vi "Select STD.vi"(8 "에러 입력(에러 없음)":errorcluster, 11 "ItemNames":string[][](array[string])) -> (0 "에러 출력":errorcluster)   [LabVIEW 2020]
uses:
  Controls/Cmd_Select Setting.ctl
  Controls/Cmd_Read Query.ctl
  Controls/Clst_Query Info.ctl
  Variables/Global_Cal STD.vi
  <vilib>/addons/database/NI_Database_API.lvlib
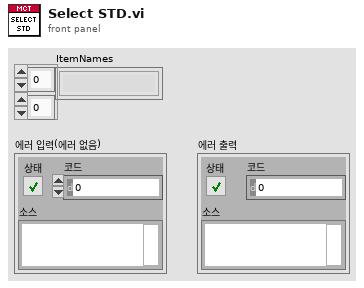
[diagram p1: front panel]
types:
  T1 = typedef "Cmd_Select Setting.ctl" = enum16{"STD Setting"}
  T2 = typedef "NI_Database_API.lvlib/Conn ObjectReference.ctl" = refnum<k1>
  T3 = typedef "Clst_Query Info.ctl" = cluster{"사번":string, "등록번호":string, "업체명":string, "세부분류코드":string, "형식":string, "기기번호":string, "FUNC":string, "FUNC_EXT":string, "옵션":string, "추가문자열":string, "일자":string, "배열 1":string[], "배열 2":string[], "항목명":string, "문자열":string, "이름":string}
  T4 = typedef "Cmd_Read Query.ctl" = enum16{"교정자 이름 얻기", "인증교정자 얻기", "기술책임자 얻기", "기책부책 얻기", "등록번호 얻기", "등록정보 얻기", "업체정보 얻기", "교정일자(CAMAS) 얻기", "교정일자(CALSTD) 얻기", "교정환경 얻기", "교정절차서 목록 얻기", "교정절차서명 얻기", "교정절차 목록얻기", "교정절차 얻기", "PROC 교정절차 얻기", "PROC SPEC 얻기", "교정절차(Func별) 얻기", "교정절차(Func_ext별) 얻기", "기관코드 얻기", "교정기능(세부분류) 얻기", "교정기능(모델) 얻기", "교정기능 목록 얻기", "교정기능 명칭 얻기", "교정기능 항목명칭 얻기", "DB (사용기준기) 얻기", "DB (기준기이름) 얻기", "DB (기준기이름목록) 얻기", "DB (기준기목록) 얻기", "DB (기준기값) 얻기", "DB (CMC) 얻기", "DB (FUNC) 얻기", "DB (CALNAME) 얻기", "DB (STDNAME) 얻기", "DB (SPEC) 얻기", "모델(항목전체) 얻기", "모델(최대범위) 얻기", "모델(최소범위) 얻기", "모델(최대최소) 얻기", "모델(범위조건) 얻기", "모델(등록요청) 얻기", "모델(형식별) 얻기", "모델(조건별) 얻기", "모델(모델검색) 얻기", "세부분류 목록 얻기", "기준기등록리스트 얻기", "STD Cal Date Check", "DB등록일자 얻기", "적용항목 얻기", "기타정보 얻기", "기준기요청 얻기", "서버버전 얻기"}
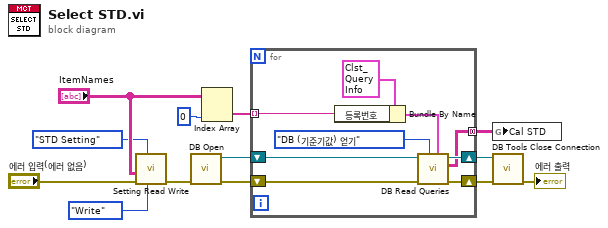
[diagram p0: block diagram]
diagram:
  n1 = call "Setting Read Write.vi"("Read/Write"=enum16{"Read", "Write"}."Write", "Select"=Cmd_Select_Setting."STD Setting", "error in (no error)"="에러 입력(에러 없음)", "Data in"="ItemNames") -> ("error out"=w10:errorcluster)  [unwired: 6 in, 1 out]
  n2 = call "DB Open.vi"("에러 입력"=w10) -> ("에러 출력"=w3:errorcluster, "참조 번호 출력"=w4:T2)  [unwired: 9 in]
  n3 = Index Array(array="ItemNames", index (col)=0 ("비활성화된 인덱스 (열)")) -> (element=w2:string[])  [unwired: 1 in]
  n4 = for {
    tunnel: w2 -> [w16] mode=indexing
    shift-right: [w20] -> w6
    shift-left: w3 -> [w22]
    shift-right: [w15] -> w5
    shift-left: w4 -> [w21]
    tunnel: [w14] -> w8 mode=concatenating
    n5 = Bundle By Name(cluster=T3 {"사번"="", "등록번호"="", "업체명"="", "세부분류코드"="", "형식"="", "기기번호"="", "FUNC"="", "FUNC_EXT"="", "옵션"="", "추가문자열"="", "일자"="", "배열 1"=[], "배열 2"=[], "항목명"="", "문자열"="", "이름"=""} ("Query info"), "등록번호"=w16) -> (w18:T3)
    n6 = call "DB Read Queries.vi"("Query info"=w18, "Query Command"=Cmd_Read_Query."DB (기준기값) 얻기", "에러 입력(에러 없음)"=w22, "참조 번호 입력"=w21) -> ("에러 출력"=w20:errorcluster, "Data"=w14:string[][], "참조 번호 출력"=w15:T2)  [unwired: 3 in, 2 out]
  }
  n7 = global write "Global_Cal STD.vi" "Cal STD"(w8) -> ()
  n8 = call <vilib>:"DB Tools Close Connection.vi"("error in (no error)"=w6, "connection reference"=w5) -> ("error out"=→"에러 출력":errorcluster)  [unwired: 5 in]
